vi "Demo - Transient Capture (Multiple Shots).vi"() -> ()   [LabVIEW 2017]
doc: "Demonstration of transient capture mode, in a continuos loop"
uses:
  Communications/Communications Library.lvlib
  GUI/Consoles/Communications Console Library.lvlib
panel:
  in  "stop":bool
  in  "ARM":bool
  in  "Soft Trigger":bool=TRUE
  out "Waveform Graph":i16[][](graph)
  in  "configuration file path":path
  in  "Pre-Trigger Samples":i32
  in  "Post-Trigger Samples":i32
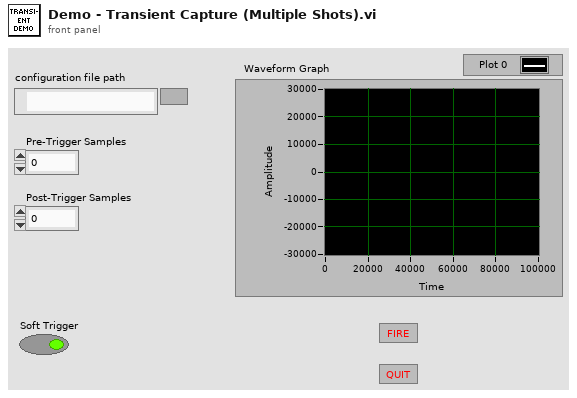
[diagram p1: front panel]
types:
  T1 = typedef "Communications Library.lvlib/DTACQ Module Carrier Configuration--Cluster.ctl" = cluster{"Name":string, "IP":string, "Control Port":i32, "Timeout (ms)":i32, "Continuous Capture Port (Multiplexed)":i32, "Start HIL Shot Port":i32, "AWG Upload Port (Multiplexed)":i32, "Download Captured Data Port (Multiplexed)":i32, "Module Slots":i32, "Module Configurations":T2[]}
  T2 = typedef "Communications Library.lvlib/DTACQ Module Configuration--Cluster.ctl" = cluster{"Name":string, "Position":string, "Module Type":T3, "Control Port":i32, "Timeout (ms)":i32, "Channels":i32}
  T3 = typedef "Communications Library.lvlib/DTACQ Device Type--Enum.ctl" = enum16{"Carrier", "Analog In Module", "Analog Out Module", "Generic Module"}
  T4 = typedef "Communications Library.lvlib/DTACQ Connection Data--Cluster.ctl" = cluster{"Description":string, "Address":string, "Port":u16, "timeout (ms)":i32, "Termination Character":string, "TCP Connection Reference":refnum<k5>, "Open Connection":bool}
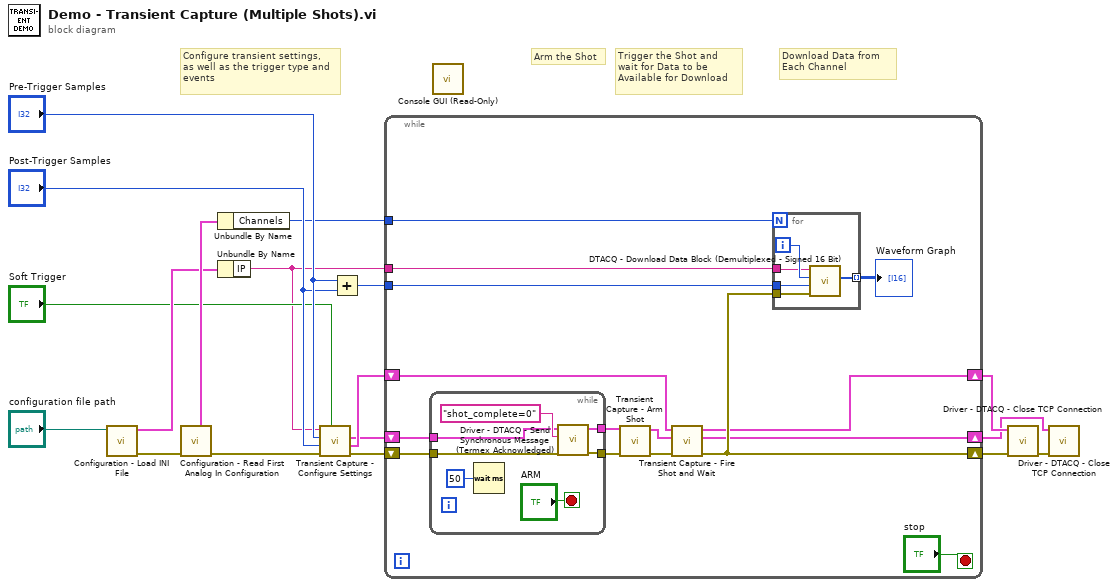
[diagram p0: block diagram]
diagram:
  # "Configure transient settings,\nas well as the trigger type and\nevents"
  # "Trigger the Shot and\nwait for Data to be\nAvailable for Download"
  # "Download Data from \nEach Channel"
  # "Arm the Shot"
  n1 = call "Configuration - Load INI File.vi"("configuration file path"="configuration file path") -> ("error out"=w14:errorcluster, "Carrier Configuration Out"=w12:T1)  [unwired: 9 in]
  n2 = call "Configuration - Read First Analog In Configuration.vi"("error in"=w14) -> ("error out"=w13:errorcluster, "AI - Module Configuration"=w15:T2)  [unwired: 6 in, 3 out]
  n3 = Unbundle By Name(w15) -> ("Channels"=w2:i32)
  n4 = Unbundle By Name(w12) -> ("IP"=w9:string)
  n5 = call "Transient Capture - Configure Settings.vi"("Soft Trigger"="Soft Trigger", "error in"=w13, "Samples to Read (Post Trigger)"="Post-Trigger Samples", "Samples to Read (Pre Trigger)"="Pre-Trigger Samples", "Address"=w9) -> ("error out"=w10:errorcluster, "AI Connection Out"=w5:T4, "Carrier Connection Out"=w1:T4)  [unwired: 4 in]
  n6 = Add(x="Pre-Trigger Samples", y="Post-Trigger Samples") -> (x+y=w8:i32)
  n7 = while {
    tunnel: w9 -> [w29]
    tunnel: w8 -> [w28]
    tunnel: w2 -> [w24]
    shift-right: [w27] -> w7
    shift-left: w10 -> [w32]
    shift-right: [w26] -> w4
    shift-left: w5 -> [w19]
    shift-right: [w25] -> w3
    shift-left: w1 -> [w23]
    stop <- "stop" stop-if-true
    n8 = while {
      tunnel: w32 -> [w38]
      tunnel: [w37] -> w31
      tunnel: w23 -> [w36]
      tunnel: [w35] -> w22
      stop <- "ARM" stop-if-true
      n9 = Wait (ms)(milliseconds to wait=u32 50) -> ()  [unwired: 1 out]
      n10 = call "Driver - DTACQ - Send Synchronous Message (Termex Acknowledged).vi"("error in"=w38, "Message to Send"="shot_complete=0", "DTACQ Connection Data In"=w36) -> ("error out"=w37:errorcluster, "DTACQ Connection Data Out"=w35:T4)  [unwired: 5 in, 2 out]
    }
    n11 = call "Transient Capture - Arm Shot.vi"("error in"=w31, "Carrier Connection Out"=w22) -> ("error out"=w30:errorcluster, "DTACQ Connection Out"=w20:T4)  [unwired: 8 in]
    n12 = call "Transient Capture - Fire Shot and Wait.vi"("error in"=w30, "Carrier Connection In"=w20, "AI Connection In"=w19) -> ("error out"=w27:errorcluster, "Carrier Connection Out"=w25:T4, "AI Connection Out"=w26:T4)  [unwired: 6 in]
    n13 = for {
      N: w24 -> [_]
      tunnel: [w44] -> w33 mode=indexing
      tunnel: w28 -> [w43]
      tunnel: w29 -> [w42]
      tunnel: w27 -> [w41]
      i -> [w45]
      n14 = call "DTACQ - Download Data Block (Demultiplexed - Signed 16 Bit).vi"("error in"=w41, "Maximum Number of Samples"=w43, "Channel Number"=w45, "Address"=w42) -> ("(Signed) 16 Bit Array"=w44:i16[])  [unwired: 5 in, 2 out]
    }
    "Waveform Graph" <- w33
  }
  n15 = call "Console GUI (Read-Only).vi"() -> ()  [unwired: 12 in]
  n16 = call "Driver - DTACQ - Close TCP Connection.vi"("error in"=w7, "DTACQ Connection Data In"=w4) -> ("error out"=w6:errorcluster)  [unwired: 8 in, 1 out]
  n17 = call "Driver - DTACQ - Close TCP Connection.vi"("error in"=w6, "DTACQ Connection Data In"=w3) -> ()  [unwired: 8 in, 2 out]
